vi "状态告警区.vi"(11 "数组":u16[](array[numeric]) format="%04xH") -> (3 "状态告警区":T1 {"工作状态" items=["空闲"=0, "水样测试"=1, "标样核查"=2, "零点核查"=3, "跨度核查"=4, "空白测试"=5, "平行样测试"=6, "加标回收"=7, "空白校准"=8, "标样校准"=9, "初始化（清洗）"=10, "调试"=22, "填充管路"=30, "清洗管路"=31, "清洗反应杯"=32]; "告警代码" items=["无告警", "缺试剂告警", "缺水样告警", "缺蒸馏水告警", "缺标液告警", "仪表漏液告警", "标定异常告警", "超量程告警", "加热异常", "低试剂预警", "超上限告警", "超下限告警", "仪表内部其他异常", "滴定异常告警", "电极异常告警", "量程切换告警", "参数设置告警", "PH电极电位异常", "电导率电极异常", "浊度光度异常", "溶解氧电极异常", "溶解氧光强异常", "温度异常告警", "PH异常告警", "溶解氧异常告警", "电导率异常告警", "浊度异常告警", "叶绿素异常告警", "藻密度异常告警", "蓝绿藻异常告警", "ORP异常告警", "氨氮异常告警", "清洁刷异常告警", "SD卡异常告警", "蓝牙异常告警", "Wifi异常告警", "流程异常告警"]; "故障代码" items=["无故障", "电机故障", "温度故障", "通讯故障", "滴定故障"]})   [LabVIEW 2016, in "斯坦道CODMn新电路板.lvlib"]
panel:
  # "共占用29 WORD"
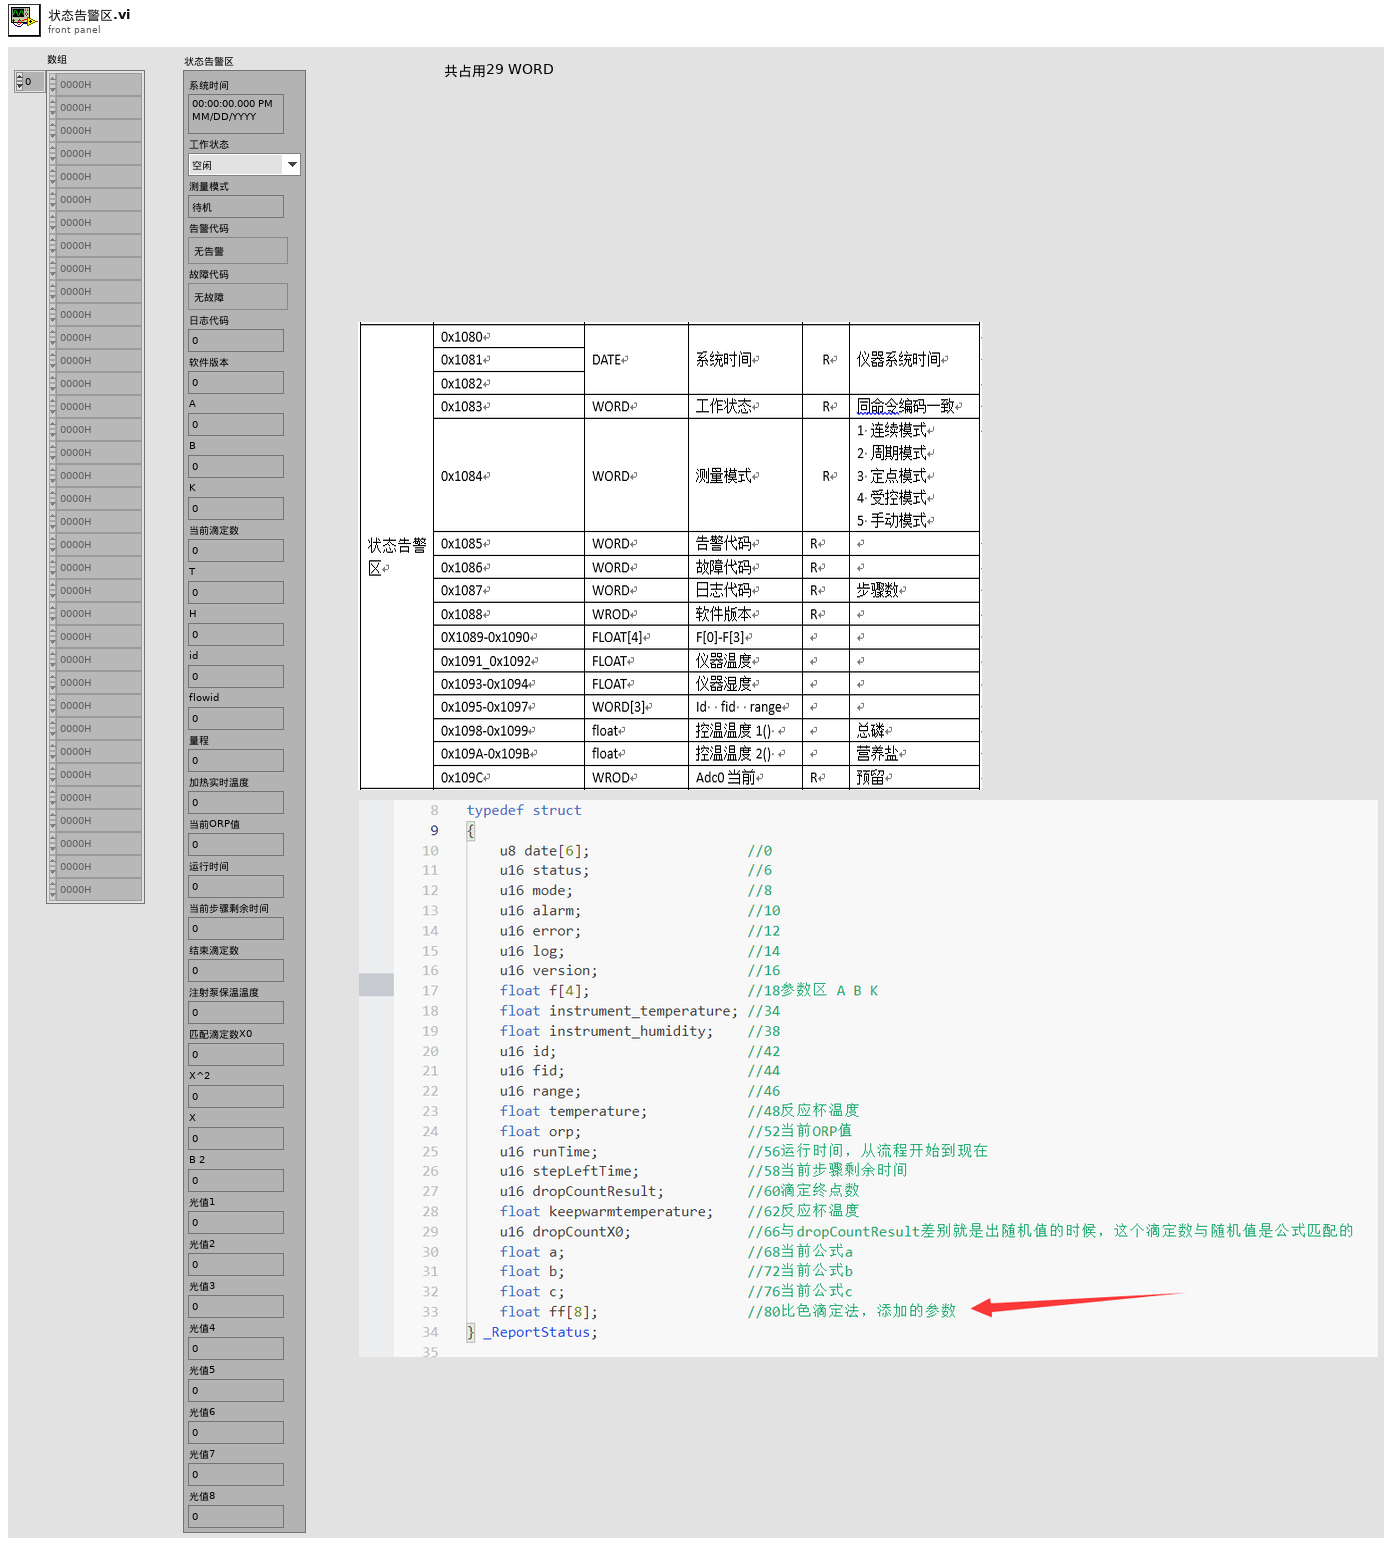
[diagram p1: front panel]
types:
  T1 = cluster{"系统时间":timestamp, "工作状态":u16, "测量模式":enum16{"待机", "连续模式", "周期模式", "定点模式", "受控模式", "手动模式"}, "告警代码":u16, "故障代码":u16, "日志代码":u16, "软件版本":u16, "A":sgl, "B":sgl, "K":sgl, "当前滴定数":sgl, "T":sgl, "H":sgl, "id":u16, "flowid":u16, "量程":u16, "加热实时温度":sgl, "当前ORP值":sgl, "运行时间":sgl, "当前步骤剩余时间":sgl, "结束滴定数":sgl, "注射泵保温温度":sgl, "匹配滴定数X0":u16, "X^2":sgl, "X":sgl, "B 2":sgl, "光值1":sgl, "光值2":sgl, "光值3":sgl, "光值4":sgl, "光值5":sgl, "光值6":sgl, "光值7":sgl, "光值8":sgl}
  T2 = cluster{"time stamp":timestamp, "WORD":u16, "WORD":u16, "WORD":u16, "WORD":u16, "WORD":u16, "WORD":u16, "FLOAT":sgl, "FLOAT":sgl, "FLOAT":sgl, "FLOAT":sgl, "FLOAT":sgl, "FLOAT":sgl, "WORD":u16, "WORD":u16, "WORD":u16, "FLOAT":sgl, "FLOAT":sgl, "WORD":u16, "WORD":u16, "WORD":u16, "FLOAT":sgl, "WORD":u16, "FLOAT":sgl, "FLOAT":sgl, "FLOAT":sgl, "FLOAT":sgl, "FLOAT":sgl, "FLOAT":sgl, "FLOAT":sgl, "FLOAT":sgl, "FLOAT":sgl, "FLOAT":sgl, "FLOAT":sgl}
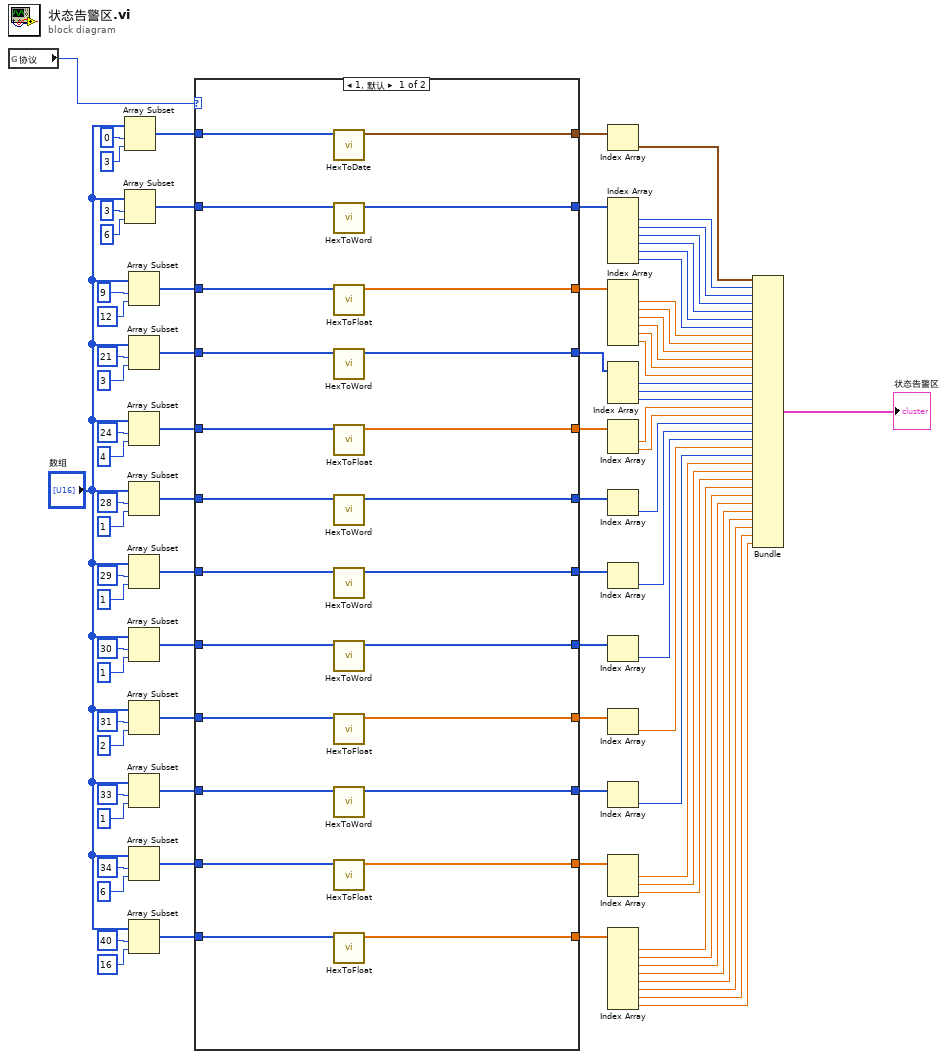
[diagram p0: block diagram]
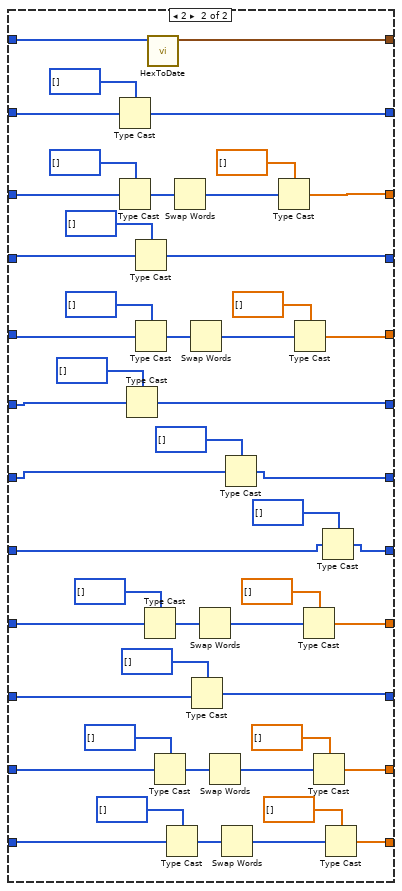
[diagram p2: hidden frame]
diagram:
  n1 = global read "CODMn断电保存全局变量.vi" "协议"() -> (w1:u16)
  n2 = Array Subset(array="数组", index=0 ("索引"), length=3 ("长度")) -> (w83:u16[])
  n3 = Array Subset(array="数组", index=3 ("索引"), length=6 ("长度")) -> (w78:u16[])
  n4 = Array Subset(array="数组", index=9 ("索引"), length=12 ("长度")) -> (w68:u16[])
  n5 = Array Subset(array="数组", index=21 ("索引"), length=3 ("索引")) -> (w58:u16[])
  n6 = Array Subset(array="数组", index=24 ("索引"), length=4 ("索引")) -> (w51:u16[])
  n7 = Array Subset(array="数组", index=28 ("索引"), length=1 ("长度")) -> (w46:u16[])
  n8 = Array Subset(array="数组", index=29 ("索引"), length=1 ("长度")) -> (w42:u16[])
  n9 = Array Subset(array="数组", index=30 ("索引"), length=1 ("长度")) -> (w35:u16[])
  n10 = Array Subset(array="数组", index=31 ("索引"), length=2 ("索引")) -> (w30:u16[])
  n11 = Array Subset(array="数组", index=33 ("索引"), length=1 ("长度")) -> (w26:u16[])
  n12 = Array Subset(array="数组", index=34 ("索引"), length=6 ("长度")) -> (w19:u16[])
  n13 = Array Subset(array="数组", index=40 ("索引"), length=16 ("长度")) -> (w14:u16[])
  n14 = case shown="1, 默认" w1 {
    tunnel: w83 -> [w109 w159]
    tunnel: [w108 w158] -> w80
    tunnel: w78 -> [w107 w150]
    tunnel: [w106 w151] -> w77
    tunnel: w68 -> [w105 w149]
    tunnel: [w104 w152] -> w67
    tunnel: w58 -> [w103 w143]
    tunnel: [w102 w142] -> w57
    tunnel: w51 -> [w101 w141]
    tunnel: [w100 w140] -> w50
    tunnel: [w99 w134] -> w47
    tunnel: w46 -> [w98 w133]
    tunnel: w42 -> [w97 w132]
    tunnel: [w96 w135] -> w41
    tunnel: [w95 w136] -> w36
    tunnel: w35 -> [w94 w131]
    tunnel: w30 -> [w93 w114]
    tunnel: [w92 w113] -> w29
    tunnel: w26 -> [w91 w111]
    tunnel: [w90 w110] -> w25
    tunnel: [w89 w117] -> w22
    tunnel: w19 -> [w88 w116]
    tunnel: w14 -> [w87 w115]
    tunnel: [w86 w118] -> w11
    frame 1, Default {
      n15 = call "HexToDate.vi"("数组"=w109) -> ("DATE"=w108:timestamp[])  [unwired: 10 in]
      n16 = call "HexToWord.vi"("数组"=w107) -> ("WORD"=w106:u16[])  [unwired: 10 in]
      n17 = call "HexToFloat.vi"("数组"=w105) -> ("FLOAT"=w104:sgl[])  [unwired: 10 in]
      n18 = call "HexToWord.vi"("数组"=w103) -> ("WORD"=w102:u16[])  [unwired: 10 in]
      n19 = call "HexToFloat.vi"("数组"=w101) -> ("FLOAT"=w100:sgl[])  [unwired: 10 in]
      n20 = call "HexToWord.vi"("数组"=w98) -> ("WORD"=w99:u16[])  [unwired: 10 in]
      n21 = call "HexToWord.vi"("数组"=w97) -> ("WORD"=w96:u16[])  [unwired: 10 in]
      n22 = call "HexToWord.vi"("数组"=w94) -> ("WORD"=w95:u16[])  [unwired: 10 in]
      n23 = call "HexToFloat.vi"("数组"=w93) -> ("FLOAT"=w92:sgl[])  [unwired: 10 in]
      n24 = call "HexToWord.vi"("数组"=w91) -> ("WORD"=w90:u16[])  [unwired: 10 in]
      n25 = call "HexToFloat.vi"("数组"=w88) -> ("FLOAT"=w89:sgl[])  [unwired: 10 in]
      n26 = call "HexToFloat.vi"("数组"=w87) -> ("FLOAT"=w86:sgl[])  [unwired: 10 in]
    }
    frame 2 {
      n27 = Type Cast(type=u16[] [], x=w150) -> (*(type *) &x=w151:u16[])
      n28 = Type Cast(type=i32[] [], x=w149) -> (*(type *) &x=w155:i32[])
      n29 = Type Cast(type=u16[] [], x=w133) -> (*(type *) &x=w134:u16[])
      n30 = Type Cast(type=u16[] [], x=w143) -> (*(type *) &x=w142:u16[])
      n31 = Type Cast(type=i32[] [], x=w141) -> (*(type *) &x=w146:i32[])
      n32 = Type Cast(type=i32[] [], x=w114) -> (*(type *) &x=w128:i32[])
      n33 = call "HexToDate.vi"("数组"=w159) -> ("DATE"=w158:timestamp[])  [unwired: 10 in]
      n34 = Type Cast(type=i32[] [], x=w116) -> (*(type *) &x=w125:i32[])
      n35 = Type Cast(type=i32[] [], x=w115) -> (*(type *) &x=w120:i32[])
      n36 = Swap Words(1:w155) -> (0:w157:i32[])
      n37 = Swap Words(1:w146) -> (0:w144:i32[])
      n38 = Type Cast(type=u16[] [], x=w111) -> (*(type *) &x=w110:u16[])
      n39 = Swap Words(1:w128) -> (0:w130:i32[])
      n40 = Swap Words(1:w125) -> (0:w123:i32[])
      n41 = Swap Words(1:w120) -> (0:w122:i32[])
      n42 = Type Cast(type=u16[] [], x=w132) -> (*(type *) &x=w135:u16[])
      n43 = Type Cast(type=sgl[] [], x=w157) -> (*(type *) &x=w152:sgl[])
      n44 = Type Cast(type=sgl[] [], x=w144) -> (*(type *) &x=w140:sgl[])
      n45 = Type Cast(type=sgl[] [], x=w130) -> (*(type *) &x=w113:sgl[])
      n46 = Type Cast(type=sgl[] [], x=w123) -> (*(type *) &x=w117:sgl[])
      n47 = Type Cast(type=u16[] [], x=w131) -> (*(type *) &x=w136:u16[])
      n48 = Type Cast(type=sgl[] [], x=w122) -> (*(type *) &x=w118:sgl[])
    }
  }
  n49 = Index Array(array=w80) -> (element=w79:timestamp)  [unwired: 1 in]
  n50 = Index Array(array=w77) -> (element #1=w76:u16, element #2=w75:u16, element #3=w74:u16, element #4=w73:u16, element #5=w72:u16, element #6=w71:u16)  [unwired: 6 in]
  n51 = Index Array(array=w67) -> (element #1=w66:sgl, element #2=w65:sgl, element #3=w64:sgl, element #4=w63:sgl, element #5=w62:sgl, element #6=w61:sgl)  [unwired: 6 in]
  n52 = Index Array(array=w57) -> (element #1=w56:u16, element #2=w55:u16, element #3=w54:u16)  [unwired: 3 in]
  n53 = Index Array(array=w50) -> (element #1=w49:sgl, element #2=w48:sgl)  [unwired: 2 in]
  n54 = Index Array(array=w47) -> (element=w44:u16)  [unwired: 1 in]
  n55 = Index Array(array=w41) -> (element=w40:u16)  [unwired: 1 in]
  n56 = Index Array(array=w36) -> (element=w33:u16)  [unwired: 1 in]
  n57 = Index Array(array=w29) -> (element=w28:sgl)  [unwired: 1 in]
  n58 = Index Array(array=w25) -> (element=w23:u16)  [unwired: 1 in]
  n59 = Index Array(array=w22) -> (element #1=w18:sgl, element #2=w16:sgl, element #3=w17:sgl)  [unwired: 3 in]
  n60 = Index Array(array=w11) -> (element #1=w9:sgl, element #2=w8:sgl, element #3=w7:sgl, element #4=w6:sgl, element #5=w5:sgl, element #6=w4:sgl, element #7=w3:sgl, element #8=w2:sgl)  [unwired: 8 in]
  n61 = Bundle("time stamp"=w79, "WORD"=w76, "WORD"=w75, "WORD"=w74, "WORD"=w73, "WORD"=w72, "WORD"=w71, "FLOAT"=w66, "FLOAT"=w65, "FLOAT"=w64, "FLOAT"=w63, "FLOAT"=w62, "FLOAT"=w61, "WORD"=w56, "WORD"=w55, "WORD"=w54, "FLOAT"=w49, "FLOAT"=w48, "WORD"=w44, "WORD"=w40, "WORD"=w33, "FLOAT"=w28, "WORD"=w23, "FLOAT"=w18, "FLOAT"=w16, "FLOAT"=w17, "FLOAT"=w9, "FLOAT"=w8, "FLOAT"=w7, "FLOAT"=w6, "FLOAT"=w5, "FLOAT"=w4, "FLOAT"=w3, "FLOAT"=w2) -> (→"状态告警区":T2)  [unwired: 1 in]
